vi "Actor Core.vi"(8 "error in":errorcluster, 11 "Chat Room in":refnum<class "Chat Room.lvclass">) -> (0 "error out":errorcluster, 3 "Actor out":refnum<class "Actor.lvclass">)   [LabVIEW 2018, in "Chat Room.lvlib" / "Chat Room.lvclass"]
doc: "(<B>Filename</B>: Actor Framework.lvlib:Actor.lvclass:Actor Core.vi)\n\nReceives messages to the actor, reacts to them, and initiates any error handling that may shut the actor down.\n\nDescendant classes may override this VI to append parallel tasks for the actor to complete while it handles messages. Overrides use the Call Parent Method node."
uses:
  Chat Room.lvclass
  C:/Program Files (x86)/National Instruments/LabVIEW 2018/vi.lib/ActorFramework/Actor/Actor.lvclass
  <vilib>/ActorFramework/Actor/Actor.lvclass
  <vilib>/ActorFramework/Actor/Actor.lvclass/Actor.ctl
  <vilib>/ActorFramework/Message Enqueuer/Message Enqueuer.lvclass/Message Enqueuer.ctl
  Chat Room.lvclass/Chat Room.ctl
  <vilib>/ActorFramework/Message Enqueuer/Init from Existing Queue.vi
  <vilib>/ActorFramework/Message Enqueuer/Enqueue.vi
  Chat Room Messages/Sine Wave Msg/Sine Wave Msg.lvclass
  C:/Program Files (x86)/National Instruments/LabVIEW 2018/vi.lib/ActorFramework/Message/Message.lvclass
  <vilib>/ActorFramework/Stop Msg/Stop Msg.lvclass
  <vilib>/ActorFramework/Message Priority Queue/Priority Enqueue.vi
  <vilib>/ActorFramework/Message Enqueuer/Message Enqueuer.lvclass
panel:
  in  "Add Error":bool
  in  "Stop":bool
  in  "Waveform Chart":dbl(graph)
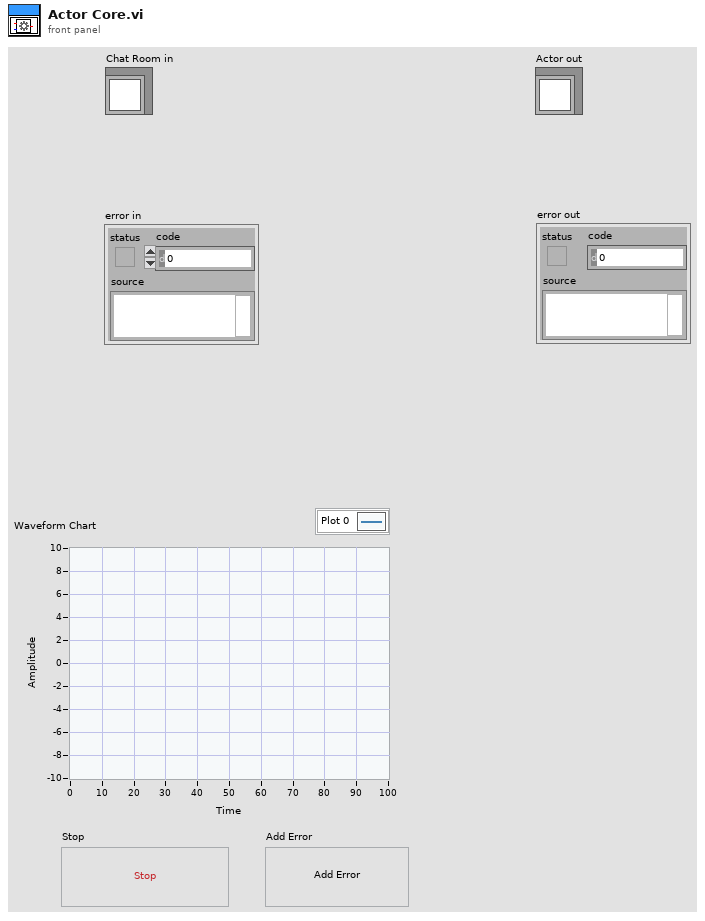
[diagram p1: front panel]
types:
  T1 = enum32{"Invalid", "Standard", "Closed", "Hidden", "Minimized", "Maximized"}
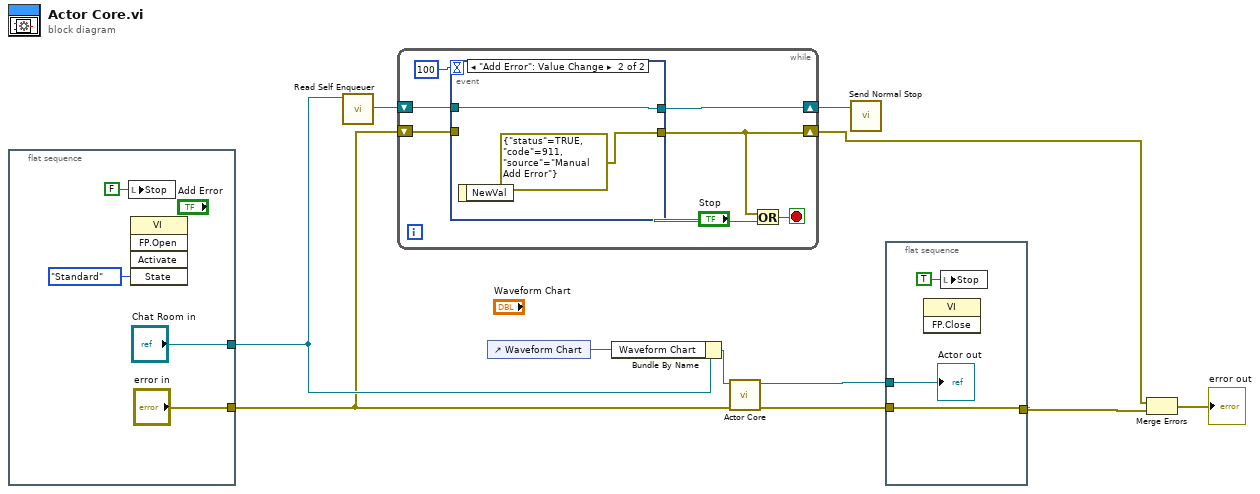
[diagram p0: block diagram]
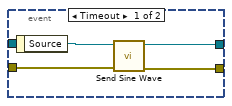
[diagram p2: hidden frame]
diagram:
  n1 = flat-sequence {
    tunnel: ["error in"] -> w5
    tunnel: ["Chat Room in"] -> w7
    frame #0 {
      n2 = local write "Stop"(FALSE ("Stop")) -> ()
      n3 = invoke class="VI" method="FP.Open"("State"=T1."Standard") -> ()  [unwired: 4 in, 5 out]
    }
  }
  n4 = call <vilib>:"Read Self Enqueuer.vi"("Actor"=w7) -> ("Self Enqueuer"=w6:refnum<class "Message Enqueuer.lvclass">)  [unwired: 10 in]
  n5 = while {
    shift-right: [w21] -> w8
    shift-left: w6 -> [w22]
    shift-right: [w20] -> w1
    shift-left: w5 -> [w16]
    stop <- w18 stop-if-true
    n6 = event shown="[1] \"Add Error\": Value Change" {
      selector: _ -> [_ _]
      dyn-events: _ -> [_ _]
      timeout: 100 -> [_ _]
      tunnel: w22 -> [w26 w28]
      tunnel: [w25 w28] -> w21
      tunnel: [w24 errorcluster {"status"=TRUE, "code"=911, "source"="Manual Add Error"} ("error out")] -> w20
      tunnel: w16 -> [w23 _]
      event Timeout {
        n7 = event-data() -> ()  [unwired: 1 in, 1 out]
        n8 = call "Send Sine Wave.vi"("error in (no error)"=w23, "Message Enqueuer"=w26) -> ("error out"=w24:errorcluster, "Message Enqueuer out"=w25:refnum<class "Message Enqueuer.lvclass">)  [unwired: 8 in]
      }
      event "Add Error": Value Change {
        n9 = event-data() -> ()  [unwired: 1 in, 1 out]
      }
    }
    n10 = Or(x=w20, y="Stop") -> (x .or. y?=w18:bool)
  }
  n11 = control-ref of="Waveform Chart"() -> (w9:refnum<vi>)
  n12 = Bundle By Name(cluster=w7, "Waveform Chart"=w9) -> (w10:refnum<class "Chat Room.lvclass">)
  n13 = call-parent "Actor Core.vi"("error in"=w5, "Actor in"=w10) -> ("error out"=w4:errorcluster, "Actor out"=w11:refnum<class "Actor.lvclass">)  [unwired: 8 in]
  n14 = call <vilib>:"Send Normal Stop.vi"("Message Enqueuer"=w8) -> ()  [unwired: 10 in, 1 out]
  n15 = flat-sequence {
    tunnel: w11 -> [w31]
    tunnel: w4 -> [w29]
    tunnel: [w29] -> w3
    frame #0 {
      n16 = invoke class="VI" method="FP.Close"() -> ()  [unwired: 3 in, 3 out]
      n17 = local write "Stop"(TRUE ("Stop")) -> ()
      "Actor out" <- w31
    }
  }
  n18 = Merge Errors(w1, w3) -> (→"error out":errorcluster)
